vi "booleanArray.vi"(1 "Array":dbl[][](array[numeric])) -> (0 "Array 2":bool[][](array[boolean]))   [LabVIEW 2014]
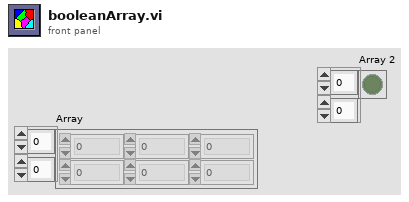
[diagram p1: front panel]
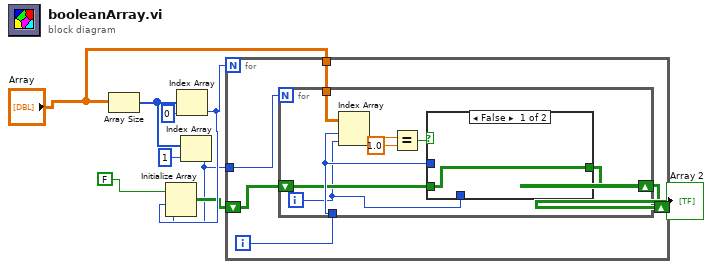
[diagram p0: block diagram]
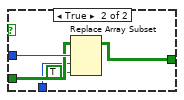
[diagram p2: hidden frame]
diagram:
  n1 = Array Size(array="Array") -> (size(s)=w9:i32[])
  n2 = Index Array(array=w9, index=0) -> (element=w5:i32)
  n3 = Index Array(array=w9, index=1) -> (element=w3:i32)
  n4 = Initialize Array(FALSE, w5, w3) -> (w4:bool[][])
  n5 = for {
    N: w5 -> [_]
    shift-right: [w13] -> w2
    shift-left: w4 -> [w14]
    tunnel: w3 -> [w12]
    tunnel: "Array" -> [w11]
    i -> [w10]
    n6 = for {
      N: w12 -> [_]
      shift-right: [w15] -> w13
      shift-left: w14 -> [w17]
      tunnel: w11 -> [w22]
      tunnel: w10 -> [w18]
      i -> [w16]
      n7 = Index Array(array=w22, index (row)=w18, index (col)=w16) -> (element=w21:dbl)
      n8 = Equal?(x=w21, y=1.0) -> (x = y?=w19:bool)
      n9 = case shown="False" w19 {
        tunnel: w18 -> [_ w28]
        tunnel: w17 -> [w23 w27]
        tunnel: w16 -> [_ w26]
        tunnel: [w23 w24] -> w15
        frame False {
        }
        frame True {
          n10 = Replace Array Subset(array=w27, new element=TRUE ("new element/subarray"), index (row)=w28, index (col)=w26) -> (w24:bool[][])
        }
      }
    }
  }
  "Array 2" <- w2
